vi "Wheel Get Value.vi"(11 "Wheel DevRef Out":T1) -> (3 "Numeric":dbl)   [LabVIEW 2015, in "Wheel.lvlib"]
doc: "Help by FRC Team 836\n\nThis VI will return the actual set parameters of wheel."
uses:
  <userlib>/836-Library/Motion_Control/Shooter_Wheel/Wheel.lvlib
  <userlib>/836-Library/Motion_Control/Shooter_Wheel/WheelControl.ctl
  <userlib>/836-Library/Motion_Control/Shooter_Wheel/Config.ctl
  <userlib>/836-Library/Motion_Control/Shooter_Wheel/Data.ctl
  <vilib>/Rock Robotics/WPI/MotorControl/WPI_MotorControlDeviceRef.ctl
  <vilib>/Rock Robotics/WPI/MotorControl/WPI_MotorControlType.ctl
  <vilib>/Rock Robotics/SystemInterfaces/DIO/FPGA_DIOPWMChannel.ctl
  <vilib>/Rock Robotics/WPI/PWM/WPI_PWMDeadband.ctl
  <vilib>/Rock Robotics/WPI/CAN/Jaguar/SubVIs/WPI_CANJaguar_ControlMode.ctl
  <vilib>/Rock Robotics/WPI/CAN/TalonSRX/WPI_CANTalonSRX_APIControlMode.ctl
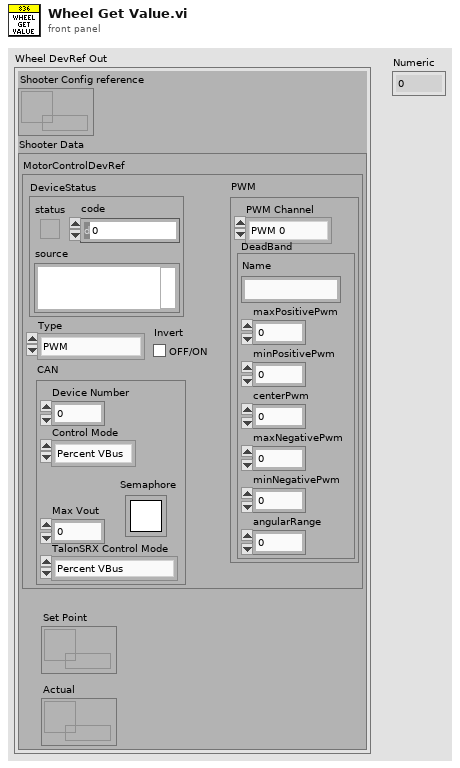
[diagram p1: front panel]
types:
  T1 = typedef "Wheel.lvlib/WheelControl.ctl" = cluster{"Shooter Config reference":refnum<data-value>, "Shooter Data":T2}
  T2 = typedef "Wheel.lvlib/Data.ctl" = cluster{"MotorControlDevRef":T3, "Set Point":refnum<k33>, "Actual":refnum<k33>}
  T3 = typedef "WPI_MotorControlDeviceRef.ctl" = cluster{"DeviceStatus":errorcluster, "Type":T4, "PWM":cluster{"PWM Channel":T5, "DeadBand":T6}, "CAN":cluster{"Device Number":u8, "Control Mode":T7, "Semaphore":T8, "Max Vout":dbl, "TalonSRX Control Mode":T9}, "Invert":bool}
  T4 = typedef "WPI_MotorControlType.ctl" = enum16{"PWM", "CAN", "CANTalonSRX"}
  T5 = typedef "FPGA_DIOPWMChannel.ctl" = enum8{"PWM 0", "PWM 1", "PWM 2", "PWM 3", "PWM 4", "PWM 5", "PWM 6", "PWM 7", "PWM 8", "PWM 9", "PWM MXP 0", "PWM MXP 1", "PWM MXP 2", "PWM MXP 3", "PWM MXP 4", "PWM MXP 5", "PWM MXP 6", "PWM MXP 7", "PWM MXP 8", "PWM MXP 9", "Invalid"}
  T6 = typedef "WPI_PWMDeadband.ctl" = cluster{"Name":string, "maxPositivePwm":i32, "minPositivePwm":i32, "centerPwm":i32, "maxNegativePwm":i32, "minNegativePwm":i32, "angularRange":u16}
  T7 = typedef "WPI_CANJaguar_ControlMode.ctl" = enum8{"Percent VBus", "Current", "Speed", "Position", "Voltage"}
  T8 = typedef "Semaphore RefNum" = refnum<k1>
  T9 = typedef "WPI_CANTalonSRX_APIControlMode.ctl" = enum8{"Percent VBus", "Speed", "Position", "Slave", "Unchanged / Invalid", "Voltage Compensation", "Current", "Motion Profile"}
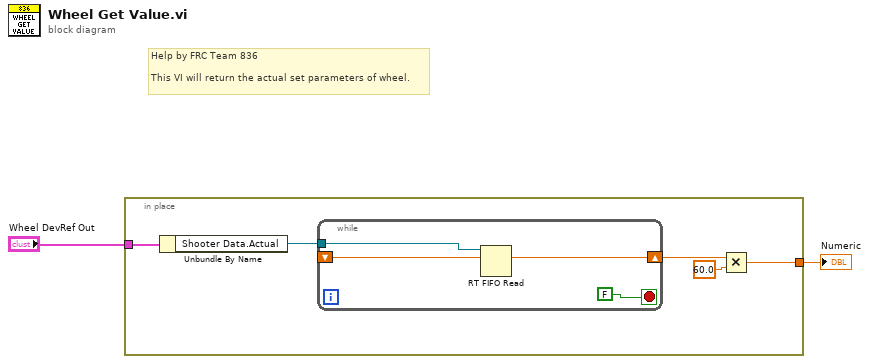
[diagram p0: block diagram]
diagram:
  # "Help by FRC Team 836\n\nThis VI will return the actual set parameters of wheel."
  n1 = in-place {
    in-place-border: "Wheel DevRef Out" -> [w7]
    in-place-border: [w5] -> w1
    n2 = Unbundle By Name(w7) -> ("Shooter Data.Actual"=w6:refnum<k33>)
    n3 = while {
      tunnel: w6 -> [w11]
      shift-right: [w9] -> w4
      shift-left: _ -> [w8]
      stop <- FALSE stop-if-true
      n4 = RT FIFO Read(0:w11, 1:w8) -> (9:w9:dbl)  [unwired: 2 in, 4 out]
    }
    n5 = Multiply(x=w4, y=60.0) -> (x*y=w5:dbl)
  }
  "Numeric" <- w1
